vi "MU Get Last Error.vi"(8 "error in (no error)":errorcluster, 11 "handle":u64) -> (0 "error out (no error)":errorcluster, 1 "lastErrorType":u32, 2 "lastError":u32, 3 "function return":u32, 5 "lastErrorText":string)   [LabVIEW 2017, in "MU_3SL_interface.lvlib"]
uses:
  MU_3SL_interface.lvlib
  lib/MU_3SL_interface.dll
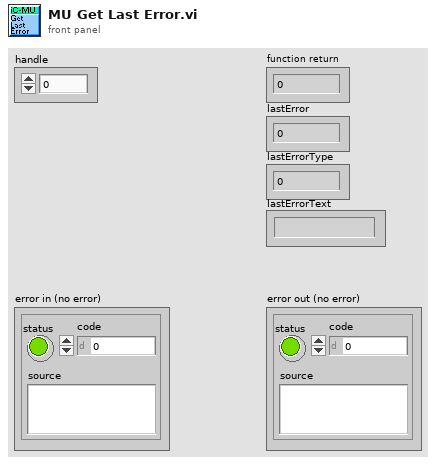
[diagram p1: front panel]
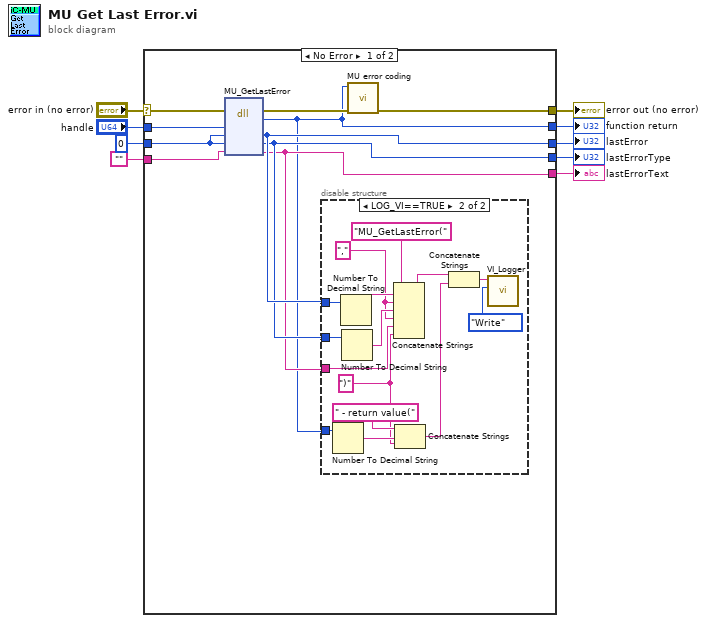
[diagram p0: block diagram]
diagram:
  n1 = case shown="No Error" "error in (no error)" {
    selector: "error in (no error)" -> [w16 w37]
    tunnel: [w10 w36] -> w9
    tunnel: "handle" -> [w19 _]
    tunnel: [w17 w37] -> w7
    tunnel: u32 0 ("pulLastError") -> [w15 w36]
    tunnel: "" -> [w14 w35]
    tunnel: [w11 w35] -> w3
    tunnel: [w13 w36] -> w2
    tunnel: [w12 w36] -> w1
    frame No Error {
      n2 = dll-call lib="C:/Users/bes/AppData/Roaming/work/mu_9so/icsubmodules/soft_mu_3sl_master/lv_interface/lib/MU_3SL_interface**.*" fn="MU_GetLastError"(error in=w16, "handle"=w19, "lastError"=w15, "lastErrorType"=w15, "lastErrorText"=w14) -> (error out=w18:errorcluster, "return type"=w10:u32, "lastError"=w13:u32, "lastErrorType"=w12:u32, "lastErrorText"=w11:string)  [unwired: 3 in, 1 out]
      n3 = disable-structure shown="LOG_VI==TRUE" {
        disable-tunnel: w10 -> [_ w32]
        disable-tunnel: w13 -> [_ w27]
        disable-tunnel: w12 -> [_ w25]
        disable-tunnel: w11 -> [_ w21]
        frame condition #0 {
        }
        frame condition #1 (active) {
          w20 = ")" ("string")
          w22 = "," ("string")
          n4 = Number To Decimal String(number=w32) -> (decimal integer string=w31:string)  [unwired: 1 in]
          n5 = Number To Decimal String(number=w27) -> (decimal integer string=w26:string)  [unwired: 1 in]
          n6 = Number To Decimal String(number=w25) -> (decimal integer string=w24:string)  [unwired: 1 in]
          n7 = Concatenate Strings("MU_GetLastError(" ("Info in"), w26, w22, w24, w22, w21, w20) -> (w30:string)
          n8 = Concatenate Strings(" - return value(" ("string"), w31, w20) -> (w29:string)
          n9 = Concatenate Strings(w30, w29) -> (w28:string)
          n10 = call "VI_Logger.vi"("Action (Read)"=enum16{"Write", "Read"}."Write", "Info in"=w28) -> ()  [unwired: 8 in, 2 out]
        }
      }
      n11 = call "MU error coding.vi"("error in (no error)"=w18, "function return in"=w10) -> ("error out"=w17:errorcluster)  [unwired: 9 in]
    }
    frame Error {
    }
  }
  "function return" <- w9
  "error out (no error)" <- w7
  "lastError" <- w2
  "lastErrorType" <- w1
  "lastErrorText" <- w3
